vi "Lockin-4461_3.0.vi"(8 "stop":bool) -> (2 "Display 1X":dbl[](graph)=[5.429724320110079e-13, -1.0557648864671476e-12, -7.674396641294021e-14, -6.653872278941454e-13, 1.3512543311352937e-12, -8.695676182925118e-13, -1.9628415610324213e-13, -4.509112104711529e-13, -1.9014266708170094e-12, 5.798774579361177e-13, -8.609700256728925e-13, 7.075652959220096e-13, 9.045027478829498e-13, -6.452533894564113e-13, 4.967470274756812e-13, 8.424888248361009e-13, 6.406927601195649e-13, -8.489816114227698e-13, 1.1065735225780592e-12, -1.952661948744721e-12, -6.717167153798251e-13, 2.170352451318973e-12, 8.533633164810356e-13, 3.230898571625721e-08, 1.4746248954003764e-12, 1.3839944130800006e-12, -1.3057445582402538e-12, -5.535836882611926e-13, -3.127772440618251e-14, -5.486152818365045e-13, -6.837509468559333e-13, -1.101009850575611e-12, -8.217908360205046e-13, 1.5919674852128345e-13, -6.878154271851141e-13, 7.351033185025182e-13, 5.704450436053545e-13, -3.500521783374724e-13, -2.9031325786509e-13, 5.361241873731532e-13, 6.133239353042052e-13, -7.509096844850103e-13, -6.782070528277833e-13, 3.6986407984691915e-13, 1.2875981278874305e-12, -9.126571382818947e-13, -1.4081682222822822e-12, 6.601643304983332e-13, 3.358604874049834e-13, 6.17891015492966e-14, 7.388961275588427e-13, -3.190507233632056e-13, 6.464810882642673e-13, -1.0585784637759772e-12, 3.1545303767551145e-13, 8.8030129738905e-13, 1.899524086368318e-12, -1.0211002590514256e-12, -8.842995728059487e-13, 4.651074986030093e-13, 0.0, 0.0, 0.0, 0.0, 0.0, 0.0, 0.0, 0.0, 0.0, 0.0, 0.0, 0.0, 0.0, 0.0, 0.0, 0.0, 0.0, 0.0, 0.0, 0.0, 0.0, 0.0, 0.0, 0.0, 0.0, 0.0, 0.0, 0.0, 0.0, 0.0, 0.0, 0.0, 0.0, 0.0, 0.0, 0.0, 0.0, 0.0, 0.0, 0.0, 0.0, 0.0, 0.0, 0.0, 0.0, 0.0, 0.0, 0.0, 0.0, 0.0, 0.0, 0.0, 0.0, 0.0, 0.0, 0.0, 0.0, 0.0, 0.0, 0.0, 0.0, 0.0, 0.0, 0.0, 0.0, 0.0, 0.0, 0.0, 0.0, 0.0, 0.0, 0.0, 0.0, 0.0, 0.0, 0.0, 0.0, 0.0, 0.0, 0.0, 0.0, 0.0, 0.0, 0.0, 0.0, 0.0, 0.0, 0.0, 0.0, 0.0, 0.0, 0.0, 0.0, 0.0, 0.0, 0.0, 0.0, 0.0, 0.0, 0.0, 0.0, 0.0, 0.0, 0.0, 0.0, 0.0, 0.0, 0.0, 0.0, 0.0, 0.0, 0.0, 0.0, 0.0, 0.0, 0.0, 0.0, 0.0, 0.0, 0.0, 0.0, 0.0, 0.0, 0.0, 0.0, 0.0, 0.0, 0.0, 0.0, 0.0, 0.0, 0.0, 0.0, 0.0, 0.0, 0.0, 0.0, 0.0, 0.0, 0.0], 3 "Input signal":dbl[][](graph))   [LabVIEW 2011]
uses:
  <vilib>/DAQmx/write.llb/DAQmx Write (Analog 1D Wfm NChan NSamp).vi
  <vilib>/DAQmx/read.llb/DAQmx Read (Analog 2D DBL NChan NSamp).vi
  DAQ-lockin-SubVI/Source/Lock-in Globles.vi
  <vilib>/DAQmx/create/channels.llb/DAQmx Create Channel (AO-Voltage-Basic).vi
  <vilib>/DAQmx/configure/timing.llb/DAQmx Timing (Sample Clock).vi
  <vilib>/DAQmx/create/channels.llb/DAQmx Create Channel (AI-Voltage-Basic).vi
  <vilib>/DAQmx/configure/trigger.llb/DAQmx Start Trigger (Digital Edge).vi
  <vilib>/DAQmx/miscellaneous.llb/DAQmx Fill In Error Info.vi
  <vilib>/Analysis/2dsp.llb/Decimate (single shot, DBL).vi
  C:/Program Files (x86)/National Instruments/LabVIEW 2011/resource/objmgr/daqmx.rc
  <vilib>/Analysis/NI_AALPro.lvlib
  <vilib>/measure/NI_MABase.lvlib
panel:
  in  "Tab Control 2":T1(tab)
  in  "Auto control  max AI rate/ AI block size":bool=TRUE
  in  "AI Buffer Size (s)":i32=50
  in  "AI Block Size":i32=20000
  out "AI Rate":dbl=26920.0 format="%.2f"
  in  "AI Configuration":T2(array[cluster])=[{"AI.Coupling"=10050, "AI.Max"=10.0, "AI.Min"=-10.0, "Input physical channels"="PXI1Slot2/ai0:1"}, {"AI.Coupling"=10050, "AI.Max"=10.0, "AI.Min"=-10.0, "Input physical channels"="PXI1Slot3/ai0:1"}] {"AI.Coupling" items=["AC"=10045, "DC"=10050, "GND"=10066]}
  in  "AO Configuration":T3(array[cluster])=[{"Output physical channels"="PXI1Slot2/ao0:1", "AO. Max"=0.1, "AO.Min"=-0.1}, {"Output physical channels"="PXI1Slot3/ao0:1", "AO. Max"=0.1, "AO.Min"=-0.1}]
  in  "OSC Configuration":T4(array[cluster])=[{"Signal Type"=enum."Sine Wave", "DC"=0.0005, "Amplitude"=0.005, "frequency"=1.346, "Phase"=0.0}, {"Signal Type"=enum."Sine Wave", "DC"=0.0, "Amplitude"=0.0, "frequency"=1.346, "Phase"=0.0}, {"Signal Type"=enum."Sine Wave", "DC"=0.0, "Amplitude"=0.0, "frequency"=1.346, "Phase"=0.0}, {"Signal Type"=enum."Sine Wave", "DC"=0.0, "Amplitude"=0.0, "frequency"=1.346, "Phase"=0.0}] {"frequency" step=0.001 format="%.3p"; "Amplitude" format="%0.2p"; "DC" min=-0.99 max=0.99 format="%.2p"}
  in  "Phase&Tc":T5(array[cluster])=[{"Phase"=0.0, "Time constant"=0.1, "Set Tc"=FALSE, "Autophase"=FALSE, "Order"=2.0}, {"Phase"=0.0, "Time constant"=0.1, "Set Tc"=FALSE, "Autophase"=FALSE, "Order"=2.0}, {"Phase"=0.0, "Time constant"=0.1, "Set Tc"=FALSE, "Autophase"=FALSE, "Order"=2.0}, {"Phase"=0.0, "Time constant"=0.1, "Set Tc"=FALSE, "Autophase"=FALSE, "Order"=2.0}] {"Phase" min=0.0 max=360.0 scale=0.0..360.0}
  in  "Amplifier Settings":u16[](array[ring])=[0, 1, 2, 3] items=["DDPCA1", "DDPCA2", "DLPVA3", "DLPVA4"]
  out "Gains":dbl[](array[numeric])=[1000000.0, 10000.0, 100.0, 100.0]
  out "Display 2":string="-  1.764176      pA"
  out "Display 1":string=" 465.107499      fA"
  in  "Tab Control":T6(tab)=enum."Input signals"
  out "Display 1Y":dbl[](graph)=[-6.015136776726478e-13, 1.035472311764227e-12, 5.188198353772234e-13, 9.334164779082207e-14, -1.5030194120082668e-12, -8.299659830246285e-13, 5.929651298804293e-13, 1.4303475305665126e-12, 1.233410917595558e-13, -4.942128189633786e-13, -5.56641126205868e-14, -1.6075217488647061e-12, -1.3472295800498274e-13, -8.683381116120352e-13, -1.3801350908965668e-12, -1.579973320066605e-12, -5.359911294273503e-13, -2.83602775541613e-13, -1.388283326074415e-13, 2.241587836500851e-12, 1.015818909665972e-12, 1.2063259781645677e-12, -7.237492590732482e-13, -2.0089800684537727e-09, -5.72873903946076e-13, 9.667067330086395e-13, -2.2804413354213683e-13, 9.302118872846608e-13, -1.7473197459755622e-13, -5.49548652613498e-13, 9.153961719844722e-14, 1.5128757165450556e-12, -1.611847036715737e-12, 1.673036083421127e-13, 1.895919985144317e-13, -2.2589321538926073e-12, 9.153463078684243e-13, 2.332390292749605e-12, 1.5850725180362008e-12, -1.2395161770271868e-12, -1.8617257075369522e-12, 8.960246859996906e-13, -4.858869389193005e-13, 8.800808803791886e-13, 1.2523505072344644e-12, 2.3323855476977413e-12, 1.7142382752330603e-12, -1.8963340507897093e-12, 1.752869886311412e-13, -3.356413093784719e-13, 2.2656871916040576e-13, 1.0273329424492362e-12, -2.1535849626269848e-13, -8.008825638107896e-13, -7.074468145745153e-14, 2.4483654170431395e-13, 8.164120676180945e-13, -1.0926978964631754e-12, -5.216842010670745e-13, -1.7641762037163097e-12, 0.0, 0.0, 0.0, 0.0, 0.0, 0.0, 0.0, 0.0, 0.0, 0.0, 0.0, 0.0, 0.0, 0.0, 0.0, 0.0, 0.0, 0.0, 0.0, 0.0, 0.0, 0.0, 0.0, 0.0, 0.0, 0.0, 0.0, 0.0, 0.0, 0.0, 0.0, 0.0, 0.0, 0.0, 0.0, 0.0, 0.0, 0.0, 0.0, 0.0, 0.0, 0.0, 0.0, 0.0, 0.0, 0.0, 0.0, 0.0, 0.0, 0.0, 0.0, 0.0, 0.0, 0.0, 0.0, 0.0, 0.0, 0.0, 0.0, 0.0, 0.0, 0.0, 0.0, 0.0, 0.0, 0.0, 0.0, 0.0, 0.0, 0.0, 0.0, 0.0, 0.0, 0.0, 0.0, 0.0, 0.0, 0.0, 0.0, 0.0, 0.0, 0.0, 0.0, 0.0, 0.0, 0.0, 0.0, 0.0, 0.0, 0.0, 0.0, 0.0, 0.0, 0.0, 0.0, 0.0, 0.0, 0.0, 0.0, 0.0, 0.0, 0.0, 0.0, 0.0, 0.0, 0.0, 0.0, 0.0, 0.0, 0.0, 0.0, 0.0, 0.0, 0.0, 0.0, 0.0, 0.0, 0.0, 0.0, 0.0, 0.0, 0.0, 0.0, 0.0, 0.0, 0.0, 0.0, 0.0, 0.0, 0.0, 0.0, 0.0, 0.0, 0.0, 0.0, 0.0, 0.0, 0.0, 0.0, 0.0]
  out "Display 2Y":dbl[](graph)=[-6.05941549125348e-10, -1.1430340211264505e-10, 1.4926553931835592e-11, 1.50809116720554e-11, -2.01455613432856e-11, 2.2500663508188414e-10, -5.53750322011223e-11, -6.325220260727363e-11, 8.972686914309565e-11, -2.1675695268903223e-10, -9.319257292382553e-11, 1.3837564135013927e-10, 3.011851516936912e-11, -1.0972720971516426e-10, -1.7192768819908462e-10, 2.1187205561264862e-10, 1.9788207965441777e-10, -2.423720638237454e-11, -2.4682239326811696e-10, -1.9335970803307808e-10, 7.039230417281883e-11, 9.011350062257116e-11, -2.665249606640579e-10, -1.453917866253117e-07, -3.0864865233522615e-10, 2.2568328220655327e-11, -1.2760612434779825e-10, 1.7406875297242865e-10, -4.880057645786918e-11, -4.660274739851506e-11, 5.7934677183048936e-11, -1.272005485436437e-10, 8.868903467098303e-11, 7.631865938582677e-11, -1.5204222349177603e-10, 1.9443492736339234e-10, -2.2100622603667065e-10, -2.363955107876496e-10, 2.553251678563293e-11, -2.8250212646006297e-10, 1.1669743589404862e-11, 2.2238028971674755e-10, 2.136484065752661e-11, 1.682371445988206e-10, 1.1620525101317565e-10, -5.560771582752512e-11, 1.2104587980470587e-10, -5.20682135443474e-11, -8.156865511367845e-11, 8.10218105283791e-11, 3.289346118088131e-11, 1.1804160110274542e-10, -5.039858478435064e-12, -1.0278298256200302e-10, -3.7448450807439117e-10, 4.9424826507365526e-11, 5.43485642775191e-11, -5.139023835896488e-11, -1.677271234483857e-11, -9.992163832446762e-11, 0.0, 0.0, 0.0, 0.0, 0.0, 0.0, 0.0, 0.0, 0.0, 0.0, 0.0, 0.0, 0.0, 0.0, 0.0, 0.0, 0.0, 0.0, 0.0, 0.0, 0.0, 0.0, 0.0, 0.0, 0.0, 0.0, 0.0, 0.0, 0.0, 0.0, 0.0, 0.0, 0.0, 0.0, 0.0, 0.0, 0.0, 0.0, 0.0, 0.0, 0.0, 0.0, 0.0, 0.0, 0.0, 0.0, 0.0, 0.0, 0.0, 0.0, 0.0, 0.0, 0.0, 0.0, 0.0, 0.0, 0.0, 0.0, 0.0, 0.0, 0.0, 0.0, 0.0, 0.0, 0.0, 0.0, 0.0, 0.0, 0.0, 0.0, 0.0, 0.0, 0.0, 0.0, 0.0, 0.0, 0.0, 0.0, 0.0, 0.0, 0.0, 0.0, 0.0, 0.0, 0.0, 0.0, 0.0, 0.0, 0.0, 0.0, 0.0, 0.0, 0.0, 0.0, 0.0, 0.0, 0.0, 0.0, 0.0, 0.0, 0.0, 0.0, 0.0, 0.0, 0.0, 0.0, 0.0, 0.0, 0.0, 0.0, 0.0, 0.0, 0.0, 0.0, 0.0, 0.0, 0.0, 0.0, 0.0, 0.0, 0.0, 0.0, 0.0, 0.0, 0.0, 0.0, 0.0, 0.0, 0.0, 0.0, 0.0, 0.0, 0.0, 0.0, 0.0, 0.0, 0.0, 0.0, 0.0, 0.0]
  out "Display 2X":dbl[](graph)=[-5.209540983663562e-10, -1.5459993952257682e-10, 1.6134503412289663e-11, 5.874866305556756e-13, 1.8940414692414204e-10, -7.864880538635719e-11, -1.175430512415376e-10, -2.923449289922303e-11, -6.392419331917415e-11, -1.8337713666585666e-10, 1.378475926172313e-10, -2.033812689548571e-10, -4.8048021398079545e-11, 7.294621415013202e-11, -6.79053402284533e-11, -7.041661428266651e-11, -1.191656553793978e-10, -3.98775872041001e-11, 1.2696913609598267e-10, -2.604239565237904e-10, 2.421076799515798e-10, -9.586074443643207e-11, -2.670963844572135e-10, 2.3385861272623584e-06, -2.9864057097814606e-10, 4.050418120279296e-11, -8.73073671365595e-11, -2.2776227141712676e-10, 1.144251733636391e-10, 2.121387219366175e-10, 3.147413611980354e-11, -2.2045845902891772e-10, -9.974235087472864e-12, 5.4453485720179784e-11, 5.028348142025519e-11, -8.026581489308628e-11, -2.006232390289361e-10, -1.4683256880763738e-11, 1.2632039237668658e-10, -6.918201795183262e-11, 7.298099701633311e-11, 1.854494343744141e-10, -4.5058253262358714e-11, 6.898844457595054e-11, 1.3404894551663646e-10, -1.269804638347461e-10, -2.584513218696582e-10, -2.0850398617076455e-10, -1.1159639123537056e-11, -2.3248834236143404e-10, -2.1026006211792789e-10, 2.970246156973531e-10, -2.6985987935710656e-10, -1.0627514528789378e-10, -2.56461698957206e-10, -4.125165616305741e-11, -1.2485179826393064e-10, -4.1504869044150744e-11, 5.037294163088094e-11, 3.015780559703068e-11, 0.0, 0.0, 0.0, 0.0, 0.0, 0.0, 0.0, 0.0, 0.0, 0.0, 0.0, 0.0, 0.0, 0.0, 0.0, 0.0, 0.0, 0.0, 0.0, 0.0, 0.0, 0.0, 0.0, 0.0, 0.0, 0.0, 0.0, 0.0, 0.0, 0.0, 0.0, 0.0, 0.0, 0.0, 0.0, 0.0, 0.0, 0.0, 0.0, 0.0, 0.0, 0.0, 0.0, 0.0, 0.0, 0.0, 0.0, 0.0, 0.0, 0.0, 0.0, 0.0, 0.0, 0.0, 0.0, 0.0, 0.0, 0.0, 0.0, 0.0, 0.0, 0.0, 0.0, 0.0, 0.0, 0.0, 0.0, 0.0, 0.0, 0.0, 0.0, 0.0, 0.0, 0.0, 0.0, 0.0, 0.0, 0.0, 0.0, 0.0, 0.0, 0.0, 0.0, 0.0, 0.0, 0.0, 0.0, 0.0, 0.0, 0.0, 0.0, 0.0, 0.0, 0.0, 0.0, 0.0, 0.0, 0.0, 0.0, 0.0, 0.0, 0.0, 0.0, 0.0, 0.0, 0.0, 0.0, 0.0, 0.0, 0.0, 0.0, 0.0, 0.0, 0.0, 0.0, 0.0, 0.0, 0.0, 0.0, 0.0, 0.0, 0.0, 0.0, 0.0, 0.0, 0.0, 0.0, 0.0, 0.0, 0.0, 0.0, 0.0, 0.0, 0.0, 0.0, 0.0, 0.0, 0.0, 0.0, 0.0]
  out "Display 3Y":dbl[](graph)=[1.0899898431091515e-10, -1.827581519364685e-12, 3.891613088455869e-11, 4.606171792041084e-11, 3.325661502628918e-12, -6.015405048742651e-12, -8.818353730362106e-11, 4.154207587561132e-11, -6.441406967923057e-11, 2.7579642959096873e-11, 2.0247087826419377e-11, -8.327687150568863e-11, 5.645080566267779e-11, -6.157569018085951e-11, 1.1122174682043351e-11, -1.1996281757831183e-11, -2.6504845634178765e-11, -7.647423208254622e-11, 6.071533763218894e-11, -1.1261384601368719e-11, -1.0198381627901654e-11, 4.1339495592751516e-11, -1.5455592976820754e-11, 2.728948705870054e-08, 6.241263230606365e-11, -8.067722846760717e-11, -2.6513314314513534e-11, 6.394988304236903e-13, 3.9796667437030913e-13, 1.8692070371173484e-11, 9.340608297065955e-11, 2.3993660602172896e-11, -9.58560062287006e-11, 3.8126603558907844e-11, 1.1951601605204586e-10, 1.2004854916369822e-11, -8.43116466469951e-11, 4.536911918648911e-11, 8.587454567532404e-12, -5.1038971112404856e-11, 6.843278254393681e-11, -3.580011760107027e-12, -1.1591384728859565e-10, -5.389281317320638e-11, 2.0343389219590334e-11, -3.787714436214173e-11, -3.9748137155015685e-12, 5.264509352400637e-11, -2.982753663474114e-11, -3.4995836799112112e-12, -3.8221570403607076e-11, -4.7570393506646275e-11, 2.1951355761018474e-11, 2.0837341666890554e-11, -5.287022087117066e-11, 2.712528172281736e-11, 5.1245525962428926e-11, -6.547691762506247e-11, 1.5121870291068263e-12, -2.2769855527826617e-11, 0.0, 0.0, 0.0, 0.0, 0.0, 0.0, 0.0, 0.0, 0.0, 0.0, 0.0, 0.0, 0.0, 0.0, 0.0, 0.0, 0.0, 0.0, 0.0, 0.0, 0.0, 0.0, 0.0, 0.0, 0.0, 0.0, 0.0, 0.0, 0.0, 0.0, 0.0, 0.0, 0.0, 0.0, 0.0, 0.0, 0.0, 0.0, 0.0, 0.0, 0.0, 0.0, 0.0, 0.0, 0.0, 0.0, 0.0, 0.0, 0.0, 0.0, 0.0, 0.0, 0.0, 0.0, 0.0, 0.0, 0.0, 0.0, 0.0, 0.0, 0.0, 0.0, 0.0, 0.0, 0.0, 0.0, 0.0, 0.0, 0.0, 0.0, 0.0, 0.0, 0.0, 0.0, 0.0, 0.0, 0.0, 0.0, 0.0, 0.0, 0.0, 0.0, 0.0, 0.0, 0.0, 0.0, 0.0, 0.0, 0.0, 0.0, 0.0, 0.0, 0.0, 0.0, 0.0, 0.0, 0.0, 0.0, 0.0, 0.0, 0.0, 0.0, 0.0, 0.0, 0.0, 0.0, 0.0, 0.0, 0.0, 0.0, 0.0, 0.0, 0.0, 0.0, 0.0, 0.0, 0.0, 0.0, 0.0, 0.0, 0.0, 0.0, 0.0, 0.0, 0.0, 0.0, 0.0, 0.0, 0.0, 0.0, 0.0, 0.0, 0.0, 0.0, 0.0, 0.0, 0.0, 0.0, 0.0, 0.0]
  out "Display 3X":dbl[](graph)=[-1.4506921493871724e-12, -2.1744765834798285e-11, -3.886449186645477e-11, -7.085075187709098e-11, -3.9703339888141896e-11, 6.618132054310167e-11, -9.271260346821464e-12, 2.7348315791542174e-12, 3.091064650959652e-11, -1.3894193780750186e-11, 7.533626719542495e-11, -6.483103188230643e-11, -5.33856411786715e-11, -2.7467380020240738e-11, -6.103708902358562e-11, -2.2007178072058763e-11, 5.834941866531552e-11, 1.1615954777255411e-11, 8.406802135603188e-11, -4.803026535071808e-11, -2.3125249162347927e-11, 2.0152063097533814e-11, 1.6224115392482473e-11, -3.1111409147652163e-07, 7.799316159585665e-11, -1.1824501871462652e-10, -2.368710541907279e-11, 1.4150563678744927e-11, 5.694824941132326e-11, -9.713715348329474e-11, 2.3131114913051142e-11, -1.8619546897619826e-11, 1.9758889124328603e-11, 2.2778491607887418e-12, -4.1834293971028396e-11, -5.885822907793353e-11, -6.035522084307104e-12, 9.06513127169592e-11, 1.9006803683115078e-12, 3.2411130907631515e-11, -2.504571126204641e-11, -1.672617800966489e-11, -2.2621410052980212e-11, 2.8752008542406313e-11, 1.4141881559218766e-10, -6.022739594210222e-11, 1.4398026519979456e-12, 1.2286212124405088e-11, -8.788648695465874e-11, -3.125736625851777e-11, 6.67849549114717e-11, -6.608662073589525e-11, -1.6367174628356684e-12, -6.139681780409842e-11, 6.804379071422838e-11, -4.089900137250954e-11, -5.2810993260533214e-11, 8.44174959623023e-12, 3.1714297415210564e-11, -2.1731790500508637e-11, 0.0, 0.0, 0.0, 0.0, 0.0, 0.0, 0.0, 0.0, 0.0, 0.0, 0.0, 0.0, 0.0, 0.0, 0.0, 0.0, 0.0, 0.0, 0.0, 0.0, 0.0, 0.0, 0.0, 0.0, 0.0, 0.0, 0.0, 0.0, 0.0, 0.0, 0.0, 0.0, 0.0, 0.0, 0.0, 0.0, 0.0, 0.0, 0.0, 0.0, 0.0, 0.0, 0.0, 0.0, 0.0, 0.0, 0.0, 0.0, 0.0, 0.0, 0.0, 0.0, 0.0, 0.0, 0.0, 0.0, 0.0, 0.0, 0.0, 0.0, 0.0, 0.0, 0.0, 0.0, 0.0, 0.0, 0.0, 0.0, 0.0, 0.0, 0.0, 0.0, 0.0, 0.0, 0.0, 0.0, 0.0, 0.0, 0.0, 0.0, 0.0, 0.0, 0.0, 0.0, 0.0, 0.0, 0.0, 0.0, 0.0, 0.0, 0.0, 0.0, 0.0, 0.0, 0.0, 0.0, 0.0, 0.0, 0.0, 0.0, 0.0, 0.0, 0.0, 0.0, 0.0, 0.0, 0.0, 0.0, 0.0, 0.0, 0.0, 0.0, 0.0, 0.0, 0.0, 0.0, 0.0, 0.0, 0.0, 0.0, 0.0, 0.0, 0.0, 0.0, 0.0, 0.0, 0.0, 0.0, 0.0, 0.0, 0.0, 0.0, 0.0, 0.0, 0.0, 0.0, 0.0, 0.0, 0.0, 0.0]
  out "Display 4Y":dbl[](graph)=[-2.8844026407170986e-11, 4.625382034220138e-11, -9.013319110948715e-11, -3.831386252102219e-11, 2.9770810866125426e-11, -1.1034670821175042e-10, 1.5257307046567804e-11, 4.8262499387874416e-11, 1.3544857909536598e-11, 1.856703050862052e-13, 2.5150436114529384e-11, -2.094748767689225e-11, -7.22408300489974e-11, -1.6319787062002432e-11, -2.6839509106935107e-11, -6.340509375775128e-11, -2.7129427161298733e-11, 4.060501667453309e-11, 8.742730286854794e-11, -7.855807339041121e-11, 3.2402653147300955e-12, -3.7221693179390055e-11, -2.721498060225258e-11, 3.163166146765944e-08, 1.9865867500357126e-11, 3.370069404127207e-11, -2.1485622596628672e-11, -1.086161315512868e-10, -1.5918432616501835e-11, -8.641508247819728e-12, -3.272966578151681e-11, -3.9968869914730473e-11, -3.7871727870708584e-11, 1.782636420557537e-11, -4.727645885793663e-12, -3.739448916633137e-11, 2.2633565117757826e-11, 3.480934154822535e-11, 7.660374794795644e-11, 4.2421105834478115e-11, -4.7175325158832496e-11, 7.467358811652501e-12, 9.053400661116483e-11, 7.680172474522351e-11, 1.9234239962884202e-11, -4.05154145894926e-11, 1.0289905284821542e-11, 1.026100591445811e-11, 2.583088099896713e-11, 4.907786066752351e-11, 5.609058148507984e-11, -3.1281978648678434e-11, -2.3787541867648086e-11, 2.931160232435559e-11, -4.803534531703235e-11, 8.40306343263819e-11, -4.556520949563492e-11, 2.7403738536690982e-11, 6.669893713819875e-11, -2.2080502155574778e-11, 0.0, 0.0, 0.0, 0.0, 0.0, 0.0, 0.0, 0.0, 0.0, 0.0, 0.0, 0.0, 0.0, 0.0, 0.0, 0.0, 0.0, 0.0, 0.0, 0.0, 0.0, 0.0, 0.0, 0.0, 0.0, 0.0, 0.0, 0.0, 0.0, 0.0, 0.0, 0.0, 0.0, 0.0, 0.0, 0.0, 0.0, 0.0, 0.0, 0.0, 0.0, 0.0, 0.0, 0.0, 0.0, 0.0, 0.0, 0.0, 0.0, 0.0, 0.0, 0.0, 0.0, 0.0, 0.0, 0.0, 0.0, 0.0, 0.0, 0.0, 0.0, 0.0, 0.0, 0.0, 0.0, 0.0, 0.0, 0.0, 0.0, 0.0, 0.0, 0.0, 0.0, 0.0, 0.0, 0.0, 0.0, 0.0, 0.0, 0.0, 0.0, 0.0, 0.0, 0.0, 0.0, 0.0, 0.0, 0.0, 0.0, 0.0, 0.0, 0.0, 0.0, 0.0, 0.0, 0.0, 0.0, 0.0, 0.0, 0.0, 0.0, 0.0, 0.0, 0.0, 0.0, 0.0, 0.0, 0.0, 0.0, 0.0, 0.0, 0.0, 0.0, 0.0, 0.0, 0.0, 0.0, 0.0, 0.0, 0.0, 0.0, 0.0, 0.0, 0.0, 0.0, 0.0, 0.0, 0.0, 0.0, 0.0, 0.0, 0.0, 0.0, 0.0, 0.0, 0.0, 0.0, 0.0, 0.0, 0.0]
  out "Display 4X":dbl[](graph)=[-1.872849874212032e-11, 1.7122412246892844e-11, -1.039280965881989e-11, -3.8219137836769534e-11, 2.54510636198968e-12, 5.649551705638675e-11, -1.2837219048125736e-11, 6.089320247177828e-11, 8.191453420346272e-12, -2.2600834935992963e-11, -5.439952919719105e-11, 5.769571050429079e-11, 1.9308897762471135e-11, -3.4192678553779385e-11, 9.300946324977131e-11, -1.727038806027537e-11, 7.995920408632173e-12, 4.071400274554549e-11, 2.268153369371362e-11, -2.0174647879223076e-11, 1.0691363677679532e-10, -1.4886887784193447e-11, -5.66145435172416e-11, -3.1370210865590164e-07, 3.490142592397077e-11, -4.99211179772148e-11, 1.3636252598244609e-11, 3.3098859041298666e-12, -1.6672726161063438e-11, 1.4892486798539355e-11, 5.223389085892288e-11, 1.9716195076308757e-11, -6.274884038088292e-11, 3.5321483840811124e-11, -7.835323866883167e-11, 1.2109030814600604e-11, 5.256527515492618e-11, 7.655498412083988e-12, -9.897929289071003e-11, 3.822872610482336e-12, 1.1209679192923232e-10, 2.9926432039962396e-11, 1.3077089526049997e-11, -4.870241767356217e-11, 2.5349979762609446e-11, 3.4612212078481696e-11, -7.616485687473168e-11, 1.7187008086182176e-11, 3.640759205650324e-12, 5.822438037809061e-11, 5.999925879620962e-11, -2.884252381395239e-11, 1.4931791499632476e-12, 2.5243703206574706e-11, -1.236460355930176e-10, 4.641707430741368e-11, -2.9998695243557e-11, -2.6680922547736572e-11, 1.4569031712088202e-11, 3.4952487260758724e-11, 0.0, 0.0, 0.0, 0.0, 0.0, 0.0, 0.0, 0.0, 0.0, 0.0, 0.0, 0.0, 0.0, 0.0, 0.0, 0.0, 0.0, 0.0, 0.0, 0.0, 0.0, 0.0, 0.0, 0.0, 0.0, 0.0, 0.0, 0.0, 0.0, 0.0, 0.0, 0.0, 0.0, 0.0, 0.0, 0.0, 0.0, 0.0, 0.0, 0.0, 0.0, 0.0, 0.0, 0.0, 0.0, 0.0, 0.0, 0.0, 0.0, 0.0, 0.0, 0.0, 0.0, 0.0, 0.0, 0.0, 0.0, 0.0, 0.0, 0.0, 0.0, 0.0, 0.0, 0.0, 0.0, 0.0, 0.0, 0.0, 0.0, 0.0, 0.0, 0.0, 0.0, 0.0, 0.0, 0.0, 0.0, 0.0, 0.0, 0.0, 0.0, 0.0, 0.0, 0.0, 0.0, 0.0, 0.0, 0.0, 0.0, 0.0, 0.0, 0.0, 0.0, 0.0, 0.0, 0.0, 0.0, 0.0, 0.0, 0.0, 0.0, 0.0, 0.0, 0.0, 0.0, 0.0, 0.0, 0.0, 0.0, 0.0, 0.0, 0.0, 0.0, 0.0, 0.0, 0.0, 0.0, 0.0, 0.0, 0.0, 0.0, 0.0, 0.0, 0.0, 0.0, 0.0, 0.0, 0.0, 0.0, 0.0, 0.0, 0.0, 0.0, 0.0, 0.0, 0.0, 0.0, 0.0, 0.0, 0.0]
  in  "Stream to disk?":bool
  in  "decimating factor":i32=400
  out "phase log":dbl[](array[numeric])=[0.999999999996331, 0.999999999996331, 0.999999999996331, 0.999999999996331]
  in  "Cancel Button":bool
  in  "Display":u16(ring) items=["X and Y", "R and Theta"]
  out "Results":dbl[][](array[numeric])=[[4.6510749860300926e-07, -1.7641762037163097e-06, 1.8244568131407326e-06, -75.23060410302357], [3.015780559703068e-07, -9.992163832446762e-07, 1.043734978041553e-06, -73.20542108368687], [-2.1731790500508636e-09, -2.276985552782662e-09, 3.147597558640707e-09, -133.6637356996649], [3.4952487260758724e-09, -2.208050215557478e-09, 4.134277374772819e-09, -32.28179248079797]]
  out "Backlog":u8(slide) scale=0.0..100.0
  out "Sampling information":cluster{"Fs":dbl, "#s":dbl}[](array[cluster])=[{"Fs"=26920.0, "#s"=20000.0}, {"Fs"=26920.0, "#s"=20000.0}]
  out "AO Task":refnum<k21>[](array[refnum])
  out "AI task":refnum<k21>[](array[refnum])
  out "Signal":dbl[][](array[numeric])
  # "Real time Adjustable Values"
  # "Configurations"
  # "Features:\n1, up to 4 lock-in amplifiers\n2, Each AO outputs an DC+AC signal, DC for sample biasing and AC for OSC. These values can be adjusted in real time.\n3, Synchronous filtering\n\nInstructions:\n1, Array index of AI configuration and AO configuration referes to board number. We have 2 PXI-4461 boards, so the max index is 1.\n2, Array number OSC configuration, Phase$&Tc control correlates to lock-in #., max index is 4.\n3, Each board can have 2 lock-in channels. Syntax for 2 channles, e.g. PXI1Slot2/ai0:1. If you want to use just one, then PXI1Slot2/ai0.\n4, Parameters (especially DC value for sample biasing) can be remotely controlled by clicking \"local\"and \"remote\" button. In real experiments, put golable values (can be found in Lock-in globles.vi) in your VI to control the lock-in and read out.\n5, choose OSC frequencies to be multiple of \nAI Rate/AI Block SIze to have best performance.\n\n-Guanglei 06/23/2011"
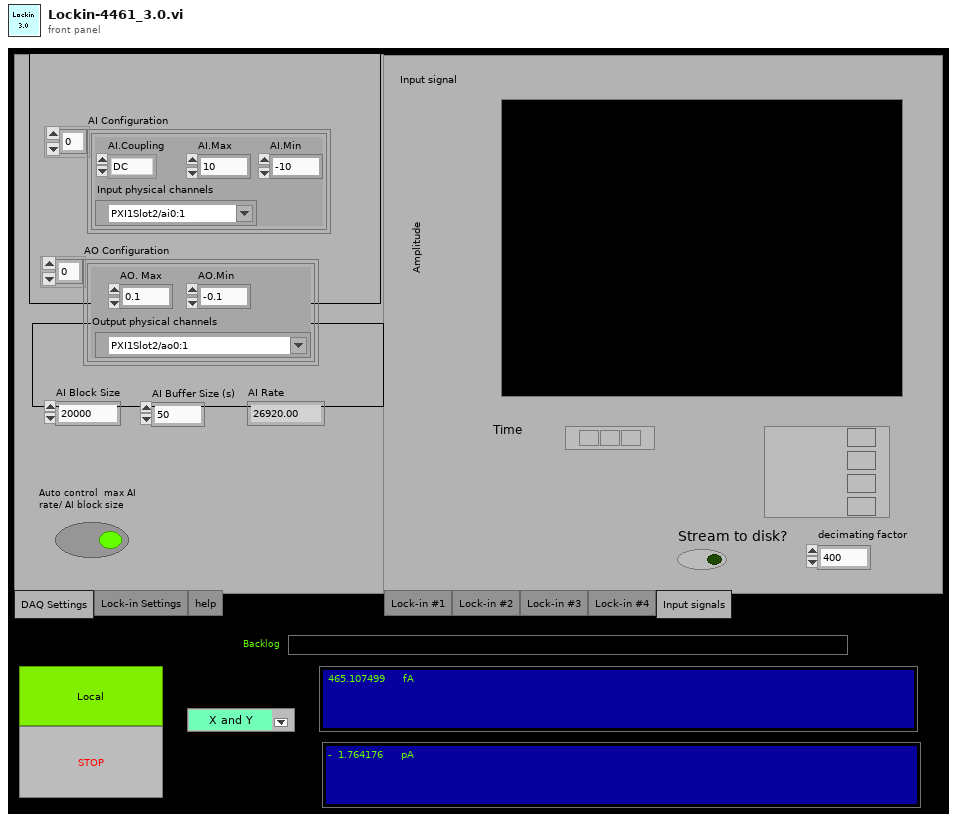
[diagram p1: front panel]
types:
  T1 = enum32{"DAQ Settings", "Lock-in Settings", "help"}
  T2 = cluster{"AI.Coupling":i32, "AI.Max":dbl, "AI.Min":dbl, "Input physical channels":tag}[]
  T3 = cluster{"Output physical channels":tag, "AO. Max":dbl, "AO.Min":dbl}[]
  T4 = cluster{"Signal Type":enum16{"Sine Wave", "Triangle Wave", "Square Wave", "Sawtooth Wave"}, "DC":dbl, "Amplitude":dbl, "frequency":dbl, "Phase":dbl}[]
  T5 = cluster{"Phase":dbl, "Time constant":dbl, "Set Tc":bool, "Autophase":bool, "Order":dbl}[]
  T6 = enum32{"Lock-in #1", "Lock-in #2", "Lock-in #3", "Lock-in #4", "Input signals"}
  T7 = cluster{"Signal Type":enum16{"Sine Wave", "Triangle Wave", "Square Wave", "Sawtooth Wave"}, "DC":dbl, "Amplitude":dbl, "frequency":dbl, "Phase":dbl}
  T8 = cluster{"AI.Coupling":i32, "AI.Max":dbl, "AI.Min":dbl, "Input physical channels":tag}
  T9 = cluster{"Output physical channels":tag, "AO. Max":dbl, "AO.Min":dbl}
  T10 = enum16{"Sine Wave", "Triangle Wave", "Square Wave", "Sawtooth Wave"}
  T11 = cluster{"Signal Type":u16, "DC":dbl, "Amplitude":dbl, "frequency":dbl, "Phase":dbl}[]
  T12 = cluster{"Signal Type":u16, "DC":dbl, "Amplitude":dbl, "frequency":dbl, "Phase":dbl}
  T13 = cluster{"Ref X":dbl[], "Ref Y":dbl[], "AI Rate":dbl, "AI Block Size":dbl, "Frequency":dbl, "Ref amp":dbl}
  T14 = cluster{"Phase":dbl, "Time constant":dbl, "Set Tc":bool, "Autophase":bool, "Order":dbl}
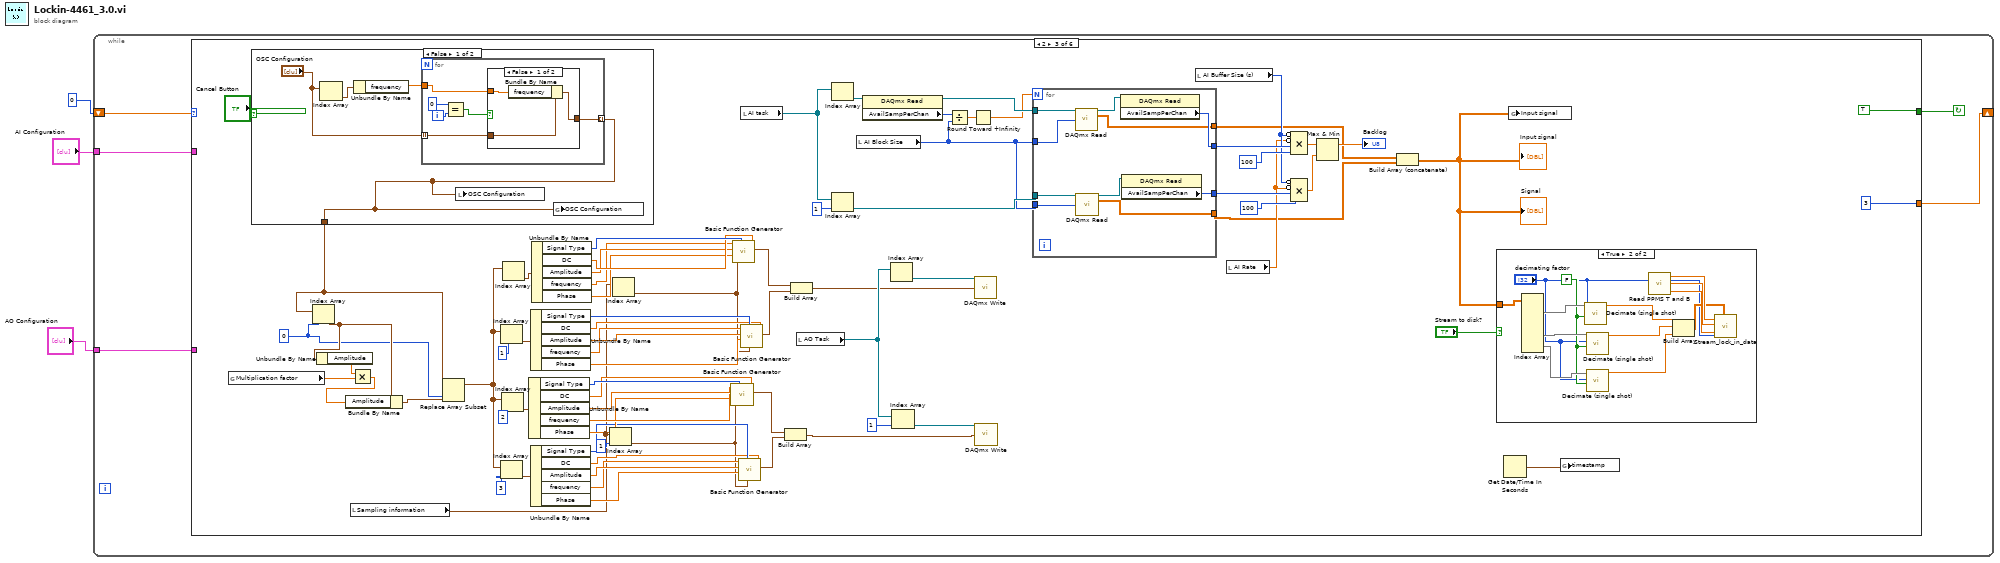
[diagram p0: block diagram]
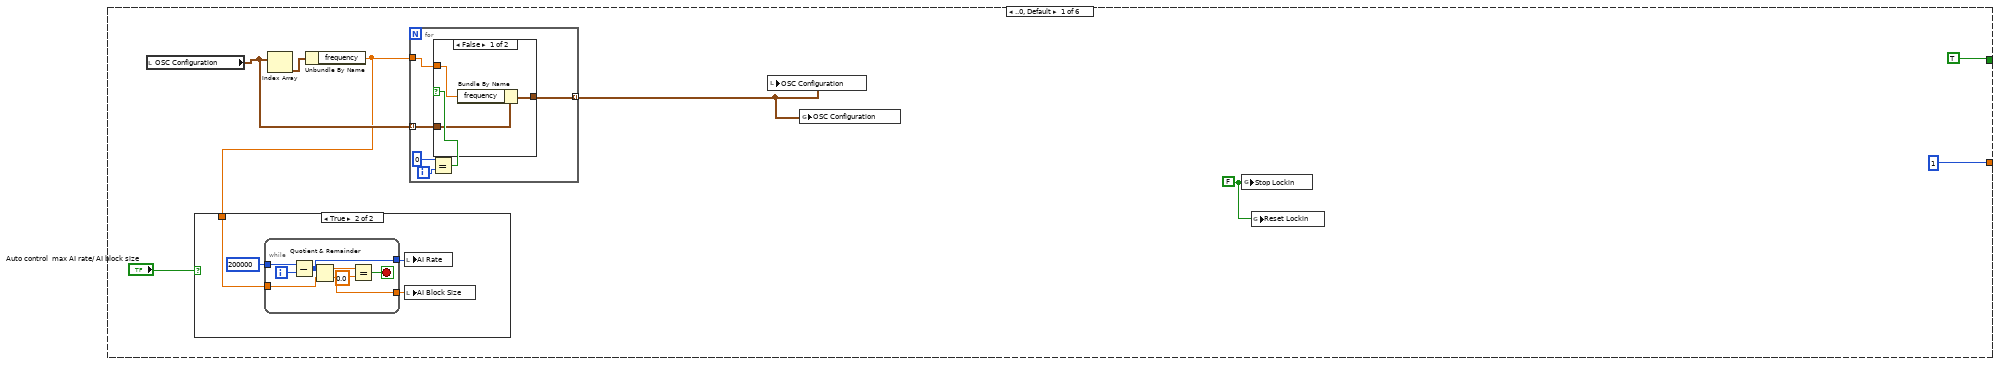
[diagram p2: hidden frame]
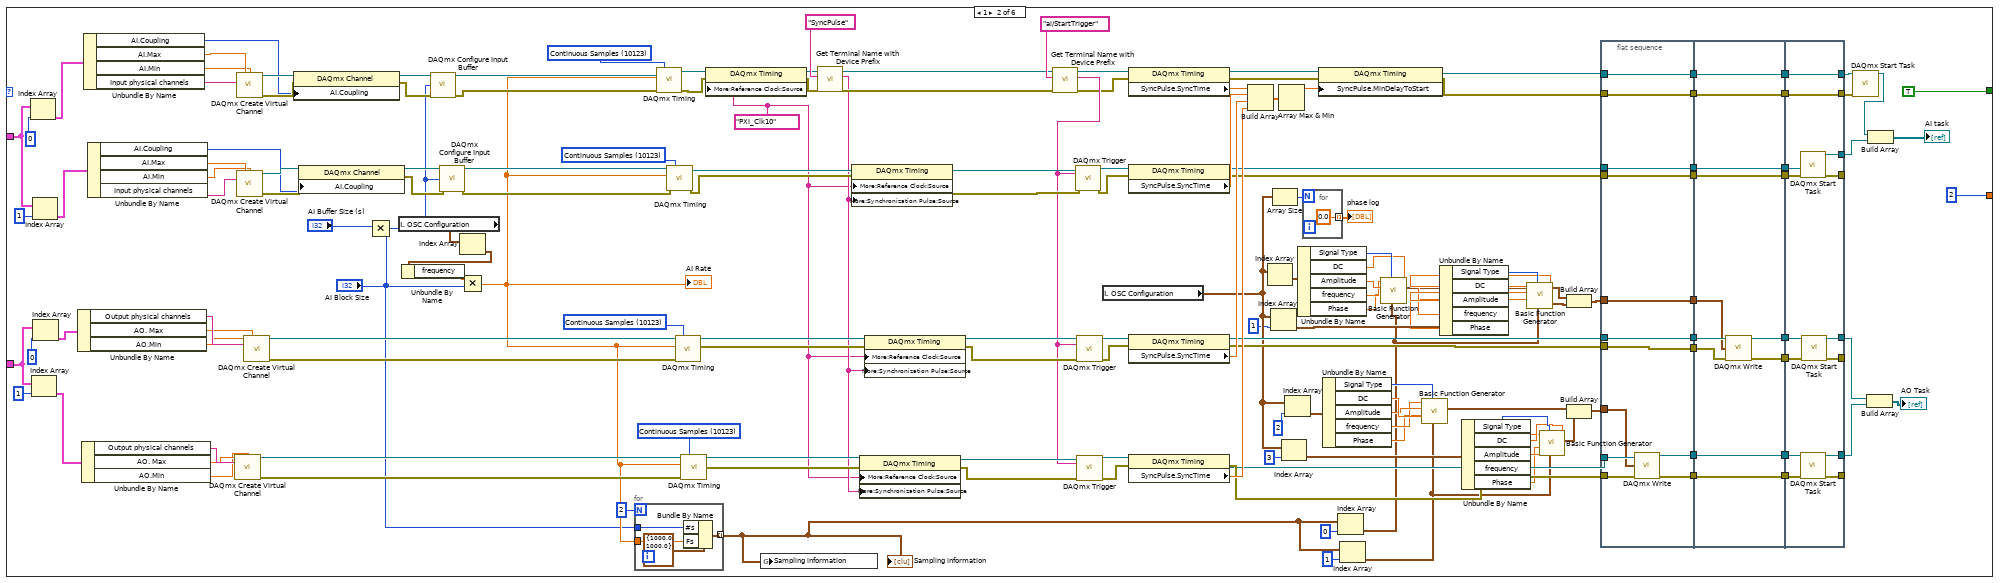
[diagram p5: hidden frame]
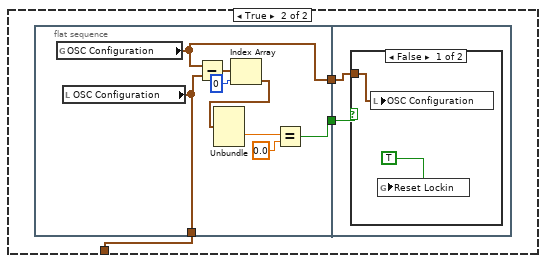
[diagram p8: hidden frame]
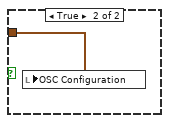
[diagram p9: hidden frame]
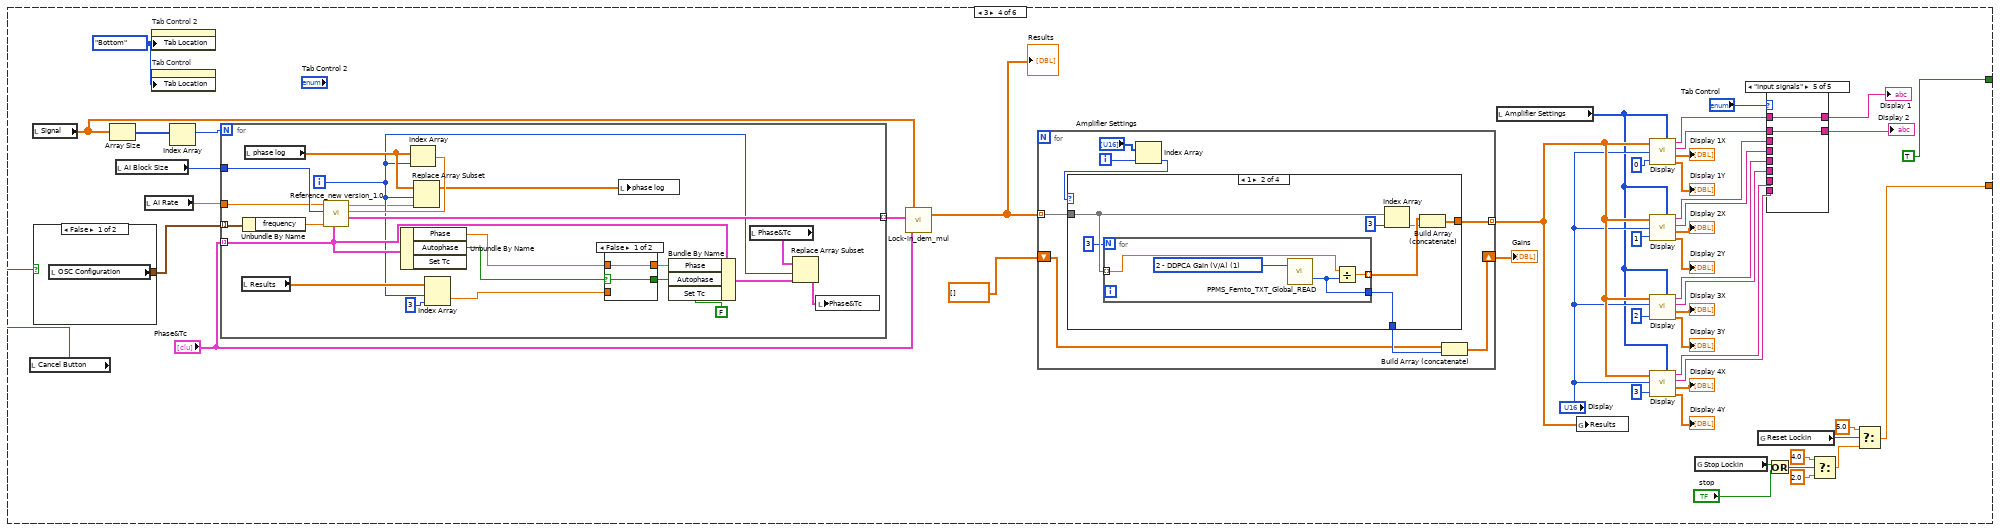
[diagram p10: hidden frame]
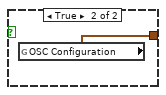
[diagram p11: hidden frame]
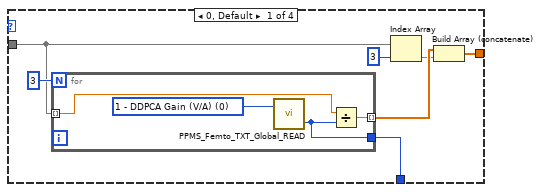
[diagram p16: hidden frame]
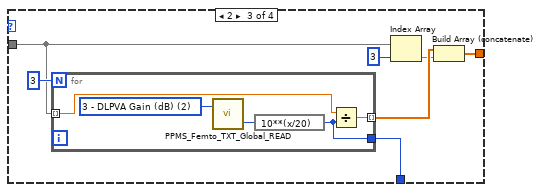
[diagram p17: hidden frame]
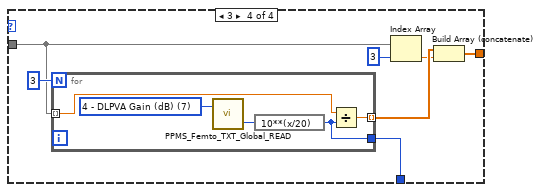
[diagram p18: hidden frame]
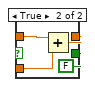
[diagram p19: hidden frame]
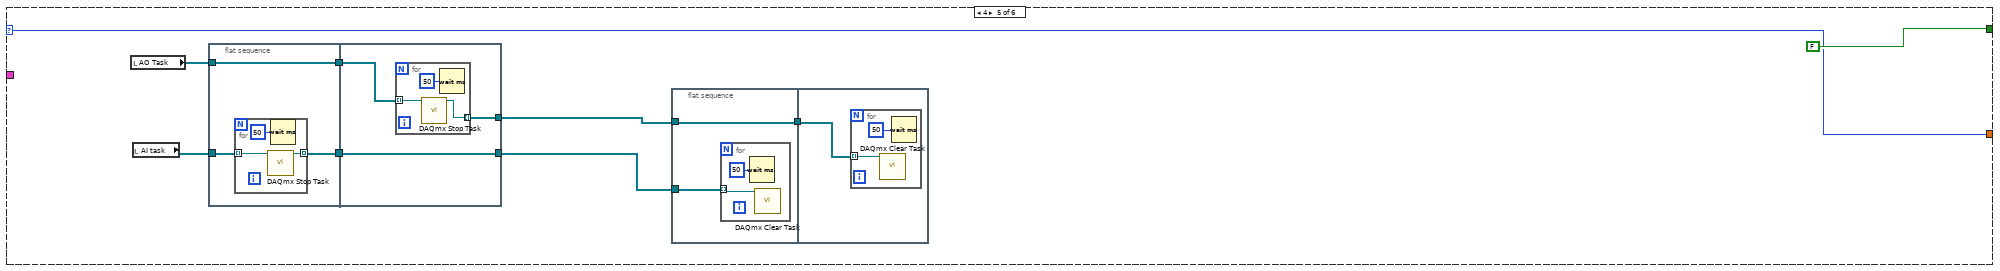
[diagram p20: hidden frame]
diagram:
  n1 = while {
    shift-right: [w8] -> _
    shift-left: 0 -> [w7]
    tunnel: "AI Configuration" -> [w6]
    tunnel: "AO Configuration" -> [w5]
    stop <- w4 continue-if-true
    n2 = case shown="2" w7 {
      selector: w7 -> [_ _ _ _ w526 _]
      tunnel: [1 2 3 w379 w526 0.0 ("f")] -> w8
      tunnel: w6 -> [_ w201 _ _ _ _]
      tunnel: w5 -> [_ w200 _ _ _ _]
      tunnel: [TRUE TRUE TRUE TRUE FALSE TRUE] -> w4
      frame ..0, Default {
        w14 = FALSE ("Stop Lockin")
        n3 = local read "OSC Configuration"() -> (w12:T4)
        n4 = Index Array(array=w12) -> (element=w13:T7)  [unwired: 1 in]
        n5 = Unbundle By Name(w13) -> ("frequency"=w11:dbl)
        n6 = case shown="True" "Auto control  max AI rate/ AI block size" {
          tunnel: w11 -> [_ w19]
          frame False {
          }
          frame True {
            n7 = while {
              tunnel: 200000 -> [w28]
              tunnel: w19 -> [w26]
              tunnel: [w22] -> w18
              tunnel: [w21] -> w17
              i -> [w27]
              stop <- w23 stop-if-true
              n8 = Subtract(x=w28, y=w27) -> (x-y=w21:i32)
              n9 = Quotient & Remainder(x=w21, y=w26) -> (x-y*floor(x/y)=w25:dbl, floor(x/y)=w22:dbl)
              n10 = Equal?(x=w25, y=0.0) -> (x = y?=w23:bool)
            }
            n11 = local write "AI Rate"(w17) -> ()
            n12 = local write "AI Block Size"(w18) -> ()
          }
        }
        n13 = for {
          tunnel: w12 -> [w31] mode=indexing
          tunnel: w11 -> [w30]
          tunnel: [w29] -> w9 mode=indexing
          i -> [w34]
          n14 = Equal?(x=0, y=w34) -> (x = y?=w32:bool)
          n15 = case shown="False" w32 {
            tunnel: w31 -> [w37 w38]
            tunnel: w30 -> [w36 _]
            tunnel: [w35 w38] -> w29
            frame False {
              n16 = Bundle By Name(cluster=w37, "frequency"=w36) -> (w35:T7)
            }
            frame True {
            }
          }
        }
        n17 = local write "OSC Configuration"(w9) -> ()
        n18 = global write "Lock-in Globles.vi" "OSC Configuration"(w9) -> ()
        n19 = global write "Lock-in Globles.vi" "Stop Lockin"(w14) -> ()
        n20 = global write "Lock-in Globles.vi" "Reset Lockin"(w14) -> ()
      }
      frame 1 {
        w108 = tag "PXI_Clk10" ("RefClk.Src")
        w166 = 10123 items=["Finite Samples"=10178, "Continuous Samples"=10123] ("sample mode")
        w167 = 10123 items=["Finite Samples"=10178, "Continuous Samples"=10123] ("sample mode")
        w174 = 10123 items=["Finite Samples"=10178, "Continuous Samples"=10123] ("sample mode")
        w175 = 10123 items=["Finite Samples"=10178, "Continuous Samples"=10123] ("sample mode")
        n21 = Index Array(array=w201, index=0) -> (element=w195:T8)
        n22 = Index Array(array=w200, index=1) -> (element=w193:T9)
        n23 = Index Array(array=w201, index=1) -> (element=w194:T8)
        n24 = Index Array(array=w200, index=0) -> (element=w192:T9)
        n25 = Unbundle By Name(w192) -> ("Output physical channels"=w117:tag, "AO. Max"=w116:dbl, "AO.Min"=w115:dbl)
        n26 = Unbundle By Name(w193) -> ("Output physical channels"=w114:tag, "AO. Max"=w113:dbl, "AO.Min"=w112:dbl)
        n27 = Unbundle By Name(w195) -> ("AI.Coupling"=w102:i32, "AI.Max"=w122:dbl, "AI.Min"=w121:dbl, "Input physical channels"=w123:tag)
        n28 = Unbundle By Name(w194) -> ("AI.Coupling"=w101:i32, "AI.Max"=w119:dbl, "AI.Min"=w118:dbl, "Input physical channels"=w120:tag)
        n29 = call-poly <vilib>:"DAQmx Create Virtual Channel.vi"("maximum value"=w113, "minimum value"=w112, "physical channels"=w114) -> ("task out"=w165:refnum<k21>, "error out"=w164:errorcluster)  [unwired: 11 in]
        n30 = call-poly <vilib>:"DAQmx Create Virtual Channel.vi"("maximum value"=w122, "minimum value"=w121, "physical channels"=w123) -> ("task out"=w106:refnum<k21>, "error out"=w105:errorcluster)  [unwired: 11 in]
        n31 = call-poly <vilib>:"DAQmx Create Virtual Channel.vi"("maximum value"=w119, "minimum value"=w118, "physical channels"=w120) -> ("task out"=w104:refnum<k21>, "error out"=w103:errorcluster)  [unwired: 11 in]
        n32 = call-poly <vilib>:"DAQmx Create Virtual Channel.vi"("maximum value"=w116, "minimum value"=w115, "physical channels"=w117) -> ("task out"=w125:refnum<k21>, "error out"=w124:errorcluster)  [unwired: 11 in]
        n33 = property class="DAQmx Channel"(reference=w106, error in=w105, "AI.Coupling"=w102) -> (reference out=w100:refnum<k21>, error out=w99:errorcluster)
        n34 = property class="DAQmx Channel"(reference=w104, error in=w103, "AI.Coupling"=w101) -> (reference out=w98:refnum<k21>, error out=w97:errorcluster)
        n35 = Multiply(x="AI Buffer Size (s)", y="AI Block Size") -> (x*y=w92:i32)
        n36 = local read "OSC Configuration"() -> (w46:T4)
        n37 = call <vilib>:"DAQmx Configure Input Buffer.vi"("task/channels in"=w100, "buffer size (in samples per channel)"=w92, "error in"=w99) -> ("task out"=w96:refnum<k21>, "error out"=w95:errorcluster)  [unwired: 11 in]
        n38 = call <vilib>:"DAQmx Configure Input Buffer.vi"("task/channels in"=w98, "buffer size (in samples per channel)"=w92, "error in"=w97) -> ("task out"=w94:refnum<k21>, "error out"=w93:errorcluster)  [unwired: 11 in]
        n39 = Index Array(array=w46) -> (element=w45:T7)  [unwired: 1 in]
        n40 = Unbundle By Name(w45) -> ("frequency"=w42:dbl)
        n41 = Multiply(x=w42, y="AI Block Size") -> (x*y=w44:dbl)
        "AI Rate" <- w44
        n42 = for {
          N: 2 -> [_]
          tunnel: w44 -> [w209]
          tunnel: "AI Block Size" -> [w208]
          tunnel: [w206] -> w64 mode=indexing
          n43 = Bundle By Name(cluster=cluster{"Fs":dbl, "#s":dbl} {"Fs"=1000.0, "#s"=1000.0} ("sampling info"), "#s"=w208, "Fs"=w209) -> (w206:cluster{"Fs":dbl, "#s":dbl})
        }
        "Sampling information" <- w64
        n44 = call-poly <vilib>:"DAQmx Timing.vi"("task/channels in"=w96, "sample mode"=w175, "rate"=w44, "error in"=w95) -> ("task out"=w169:refnum<k21>, "error out"=w168:errorcluster)  [unwired: 10 in]
        n45 = call-poly <vilib>:"DAQmx Timing.vi"("task/channels in"=w94, "sample mode"=w174, "rate"=w44, "error in"=w93) -> ("task out"=w171:refnum<k21>, "error out"=w170:errorcluster)  [unwired: 10 in]
        n46 = call-poly <vilib>:"DAQmx Timing.vi"("task/channels in"=w125, "sample mode"=w167, "rate"=w44, "error in"=w124) -> ("task out"=w162:refnum<k21>, "error out"=w161:errorcluster)  [unwired: 10 in]
        n47 = call-poly <vilib>:"DAQmx Timing.vi"("task/channels in"=w165, "sample mode"=w166, "rate"=w44, "error in"=w164) -> ("task out"=w163:refnum<k21>, "error out"=w158:errorcluster)  [unwired: 10 in]
        n48 = property class="DAQmx Timing"(reference=w169, error in=w168, "More:Reference Clock:Source"=w108) -> (reference out=w109:refnum<k21>, error out=w107:errorcluster)
        n49 = global write "Lock-in Globles.vi" "Sampling information"(w64) -> ()
        n50 = call "Get Terminal Name with Device Prefix.vi"("error in (no error)"=w107, "Local Terminal Name"="SyncPulse", "task/channels in"=w109) -> ("error out"=w151:errorcluster, "Terminal Name with Device Prefix"=w110:tag, "task out"=w152:refnum<k21>)  [unwired: 6 in]
        n51 = property class="DAQmx Timing"(reference=w171, error in=w170, "More:Reference Clock:Source"=w108, "More:Synchronization Pulse:Source"=w110) -> (reference out=w173:refnum<k21>, error out=w172:errorcluster)
        n52 = property class="DAQmx Timing"(reference=w163, error in=w158, "More:Reference Clock:Source"=w108, "More:Synchronization Pulse:Source"=w110) -> (reference out=w155:refnum<k21>, error out=w154:errorcluster)
        n53 = property class="DAQmx Timing"(reference=w162, error in=w161, "More:Reference Clock:Source"=w108, "More:Synchronization Pulse:Source"=w110) -> (reference out=w157:refnum<k21>, error out=w156:errorcluster)
        n54 = call "Get Terminal Name with Device Prefix.vi"("error in (no error)"=w151, "Local Terminal Name"="ai/StartTrigger", "task/channels in"=w152) -> ("error out"=w148:errorcluster, "Terminal Name with Device Prefix"=w150:tag, "task out"=w149:refnum<k21>)  [unwired: 6 in]
        n55 = call-poly <vilib>:"DAQmx Trigger.vi"("task/channels in"=w173, "source"=w150, "error in"=w172) -> ("task out"=w144:refnum<k21>, "error out"=w145:errorcluster)  [unwired: 11 in]
        n56 = call-poly <vilib>:"DAQmx Trigger.vi"("task/channels in"=w157, "source"=w150, "error in"=w156) -> ("task out"=w142:refnum<k21>, "error out"=w143:errorcluster)  [unwired: 11 in]
        n57 = call-poly <vilib>:"DAQmx Trigger.vi"("task/channels in"=w155, "source"=w150, "error in"=w154) -> ("task out"=w147:refnum<k21>, "error out"=w146:errorcluster)  [unwired: 11 in]
        n58 = local read "OSC Configuration"() -> (w65:T4)
        n59 = property class="DAQmx Timing"(reference=w149, error in=w148) -> (reference out=w139:refnum<k21>, error out=w140:errorcluster, "SyncPulse.SyncTime"=w141:dbl)
        n60 = property class="DAQmx Timing"(reference=w144, error in=w145) -> (reference out=w130:refnum<k21>, error out=w131:errorcluster, "SyncPulse.SyncTime"=w136:dbl)
        n61 = property class="DAQmx Timing"(reference=w142, error in=w143) -> (reference out=w128:refnum<k21>, error out=w129:errorcluster, "SyncPulse.SyncTime"=w135:dbl)
        n62 = property class="DAQmx Timing"(reference=w147, error in=w146) -> (reference out=w126:refnum<k21>, error out=w127:errorcluster, "SyncPulse.SyncTime"=w134:dbl)
        n63 = Build Array(w141, w136, w135, w134) -> (w138:dbl[])
        n64 = Index Array(array=w65) -> (element=w88:T7)  [unwired: 1 in]
        n65 = Index Array(array=w65, index=1) -> (element=w87:T7)
        n66 = Array Size(array=w65) -> (size(s)=w202:i32)
        n67 = Array Max & Min(array=w138) -> (max value=w137:dbl)  [unwired: 3 out]
        n68 = Index Array(array=w65, index=3) -> (element=w86:T7)
        n69 = Index Array(array=w65, index=2) -> (element=w89:T7)
        n70 = Unbundle By Name(w88) -> ("Signal Type"=w85:T10, "DC"=w84:dbl, "Amplitude"=w83:dbl, "frequency"=w82:dbl, "Phase"=w81:dbl)
        n71 = for {
          N: w202 -> [_]
          tunnel: [0.0] -> w203 mode=indexing
        }
        "phase log" <- w203
        n72 = property class="DAQmx Timing"(reference=w139, error in=w140, "SyncPulse.MinDelayToStart"=w137) -> (reference out=w132:refnum<k21>, error out=w133:errorcluster)
        n73 = Unbundle By Name(w89) -> ("Signal Type"=w75:T10, "DC"=w74:dbl, "Amplitude"=w73:dbl, "frequency"=w72:dbl, "Phase"=w71:dbl)
        n74 = Index Array(array=w64, index=0) -> (element=w61:cluster{"Fs":dbl, "#s":dbl})
        n75 = Index Array(array=w64, index=1) -> (element=w60:cluster{"Fs":dbl, "#s":dbl})
        n76 = call <vilib>:"Basic Function Generator.vi"("offset"=w84, "sampling info"=w61, "signal type"=w85, "phase"=w81, "amplitude"=w83, "frequency"=w82) -> ("signal out"=w59:waveform(dbl))  [unwired: 3 in, 2 out]
        n77 = call <vilib>:"Basic Function Generator.vi"("offset"=w74, "sampling info"=w60, "signal type"=w75, "phase"=w71, "amplitude"=w73, "frequency"=w72) -> ("signal out"=w55:waveform(dbl))  [unwired: 3 in, 2 out]
        n78 = Unbundle By Name(w87) -> ("Signal Type"=w80:T10, "DC"=w79:dbl, "Amplitude"=w78:dbl, "frequency"=w77:dbl, "Phase"=w76:dbl)
        n79 = Unbundle By Name(w86) -> ("Signal Type"=w70:T10, "DC"=w69:dbl, "Amplitude"=w68:dbl, "frequency"=w67:dbl, "Phase"=w66:dbl)
        n80 = call <vilib>:"Basic Function Generator.vi"("offset"=w79, "sampling info"=w61, "signal type"=w80, "phase"=w76, "amplitude"=w78, "frequency"=w77) -> ("signal out"=w58:waveform(dbl))  [unwired: 3 in, 2 out]
        n81 = call <vilib>:"Basic Function Generator.vi"("offset"=w69, "sampling info"=w60, "signal type"=w70, "phase"=w66, "amplitude"=w68, "frequency"=w67) -> ("signal out"=w54:waveform(dbl))  [unwired: 3 in, 2 out]
        n82 = Build Array(w59, w58) -> (w57:waveform(dbl)[])
        n83 = Build Array(w55, w54) -> (w53:waveform(dbl)[])
        n84 = flat-sequence {
          tunnel: w133 -> [w218]
          tunnel: w132 -> [w219]
          tunnel: w131 -> [w220]
          tunnel: w130 -> [w221]
          tunnel: [w221] -> w191
          tunnel: [w220] -> w190
          tunnel: [w219] -> w189
          tunnel: [w218] -> w188
          tunnel: [w217] -> w187
          tunnel: w129 -> [w217]
          tunnel: [w216] -> w186
          tunnel: w128 -> [w216]
          tunnel: w127 -> [w215]
          tunnel: w126 -> [w214]
          tunnel: [w213] -> w185
          tunnel: [w212] -> w184
          tunnel: w57 -> [w211]
          tunnel: [w211] -> w56
          tunnel: w53 -> [w210]
          tunnel: [w232] -> w183
          tunnel: [w231] -> w182
          tunnel: [w230] -> w181
          tunnel: [w229] -> w180
          tunnel: w191 -> [w232]
          tunnel: w190 -> [w231]
          tunnel: w189 -> [w230]
          tunnel: w188 -> [w229]
          tunnel: w187 -> [w228]
          tunnel: w186 -> [w227]
          tunnel: [w226] -> w179
          tunnel: w185 -> [w226]
          tunnel: [w225] -> w178
          tunnel: w184 -> [w225]
          tunnel: [w224] -> w177
          tunnel: [w223] -> w176
          tunnel: w56 -> [w222]
          tunnel: [w239] -> _
          tunnel: [w240] -> w49
          tunnel: [w241] -> _
          tunnel: [w242] -> w48
          tunnel: [w243] -> _
          tunnel: [w245] -> w51
          tunnel: [w238] -> w160
          tunnel: [w237] -> w159
          tunnel: w183 -> [w246]
          tunnel: w182 -> [w244]
          tunnel: w181 -> [w238]
          tunnel: w180 -> [w237]
          tunnel: w179 -> [w236]
          tunnel: w178 -> [w235]
          tunnel: w177 -> [w234]
          tunnel: w176 -> [w233]
          frame #0 {
            n85 = call-poly <vilib>:"DAQmx Write.vi"("task/channels in"=w214, "data"=w210, "error in"=w215) -> ("task out"=w212:refnum<k21>, "error out"=w213:errorcluster)  [unwired: 10 in, 1 out]
          }
          frame #1 {
            n86 = call-poly <vilib>:"DAQmx Write.vi"("task/channels in"=w227, "data"=w222, "error in"=w228) -> ("task out"=w223:refnum<k21>, "error out"=w224:errorcluster)  [unwired: 10 in, 1 out]
          }
          frame #2 {
            n87 = call <vilib>:"DAQmx Start Task.vi"("task/channels in"=w246, "error in"=w244) -> ("task out"=w245:refnum<k21>, "error out"=w243:errorcluster)  [unwired: 12 in]
            n88 = call <vilib>:"DAQmx Start Task.vi"("task/channels in"=w235, "error in"=w236) -> ("task out"=w242:refnum<k21>, "error out"=w241:errorcluster)  [unwired: 12 in]
            n89 = call <vilib>:"DAQmx Start Task.vi"("task/channels in"=w233, "error in"=w234) -> ("task out"=w240:refnum<k21>, "error out"=w239:errorcluster)  [unwired: 12 in]
          }
        }
        n90 = call <vilib>:"DAQmx Start Task.vi"("task/channels in"=w160, "error in"=w159) -> ("task out"=w52:refnum<k21>)  [unwired: 12 in, 1 out]
        n91 = Build Array(w49, w48) -> (→"AO Task":refnum<k21>[])
        n92 = Build Array(w52, w51) -> (→"AI task":refnum<k21>[])
      }
      frame 2 {
        w312 = 0 ("index")
        n93 = global read "Lock-in Globles.vi" "Multiplication factor"() -> (w316:dbl)
        n94 = case shown="False" "Cancel Button" {
          tunnel: [w346 w362] -> w313
          frame False {
            n95 = Index Array(array="OSC Configuration") -> (element=w349:T7)  [unwired: 1 in]
            n96 = Unbundle By Name(w349) -> ("frequency"=w348:dbl)
            n97 = for {
              tunnel: "OSC Configuration" -> [w352] mode=indexing
              tunnel: w348 -> [w351]
              tunnel: [w350] -> w346 mode=indexing
              i -> [w355]
              n98 = Equal?(x=0, y=w355) -> (x = y?=w353:bool)
              n99 = case shown="False" w353 {
                tunnel: w352 -> [w358 w359]
                tunnel: w351 -> [w357 _]
                tunnel: [w356 w359] -> w350
                frame False {
                  n100 = Bundle By Name(cluster=w358, "frequency"=w357) -> (w356:T7)
                }
                frame True {
                }
              }
            }
            n101 = local write "OSC Configuration"(w346) -> ()
            n102 = global write "Lock-in Globles.vi" "OSC Configuration"(w346) -> ()
          }
          frame True {
            n103 = flat-sequence {
              tunnel: [w365] -> w362
              tunnel: [w364] -> w361
              tunnel: [w363] -> w360
              tunnel: w361 -> [w372]
              tunnel: w360 -> [w371]
              frame #0 {
                n104 = global read "Lock-in Globles.vi" "OSC Configuration"() -> (w364:T4)
                n105 = local read "OSC Configuration"() -> (w365:T4)
                n106 = Subtract(x=w364, y=w365) -> (x-y=w370:T11)
                n107 = Index Array(array=w370, index=0) -> (element=w368:T12)
                n108 = Unbundle(w368) -> ("frequency"=w367:dbl)  [unwired: 4 out]
                n109 = Equal?(x=w367, y=0.0) -> (x = y?=w363:bool)
              }
              frame #1 {
                n110 = case shown="False" w371 {
                  tunnel: w372 -> [w374 w375]
                  frame False {
                    n111 = local write "OSC Configuration"(w374) -> ()
                    n112 = global write "Lock-in Globles.vi" "Reset Lockin"(TRUE ("Reset Lockin")) -> ()
                  }
                  frame True {
                    n113 = local write "OSC Configuration"(w375) -> ()
                  }
                }
              }
            }
          }
        }
        n114 = Index Array(array=w313, index=w312) -> (element=w317:T7)
        n115 = Unbundle By Name(w317) -> ("Amplitude"=w315:dbl)
        n116 = local read "Sampling information"() -> (w251:cluster{"Fs":dbl, "#s":dbl}[])
        n117 = Multiply(x=w315, y=w316) -> (x*y=w314:dbl)
        n118 = Bundle By Name(cluster=w317, "Amplitude"=w314) -> (w311:T7)
        n119 = Replace Array Subset(array=w313, new element=w311, index=w312) -> (w272:T4)
        n120 = Index Array(array=w272, index=1) -> (element=w284:T7)
        n121 = Index Array(array=w272, index=3) -> (element=w268:T7)
        n122 = Index Array(array=w272, index=2) -> (element=w269:T7)
        n123 = Index Array(array=w272) -> (element=w285:T7)  [unwired: 1 in]
        n124 = Unbundle By Name(w269) -> ("Signal Type"=w267:T10, "DC"=w266:dbl, "Amplitude"=w265:dbl, "frequency"=w264:dbl, "Phase"=w263:dbl)
        n125 = Unbundle By Name(w284) -> ("Signal Type"=w278:T10, "DC"=w277:dbl, "Amplitude"=w276:dbl, "frequency"=w275:dbl, "Phase"=w274:dbl)
        n126 = Unbundle By Name(w268) -> ("Signal Type"=w262:T10, "DC"=w261:dbl, "Amplitude"=w260:dbl, "frequency"=w259:dbl, "Phase"=w258:dbl)
        n127 = Unbundle By Name(w285) -> ("Signal Type"=w283:T10, "DC"=w282:dbl, "Amplitude"=w281:dbl, "frequency"=w280:dbl, "Phase"=w279:dbl)
        n128 = Index Array(array=w251, index=1) -> (element=w255:cluster{"Fs":dbl, "#s":dbl})
        n129 = Index Array(array=w251) -> (element=w256:cluster{"Fs":dbl, "#s":dbl})  [unwired: 1 in]
        n130 = call <vilib>:"Basic Function Generator.vi"("offset"=w266, "sampling info"=w255, "signal type"=w267, "phase"=w263, "amplitude"=w265, "frequency"=w264) -> ("signal out"=w254:waveform(dbl))  [unwired: 3 in, 2 out]
        n131 = call <vilib>:"Basic Function Generator.vi"("offset"=w282, "sampling info"=w256, "signal type"=w283, "phase"=w279, "amplitude"=w281, "frequency"=w280) -> ("signal out"=w288:waveform(dbl))  [unwired: 3 in, 2 out]
        n132 = call <vilib>:"Basic Function Generator.vi"("offset"=w261, "sampling info"=w255, "signal type"=w262, "phase"=w258, "amplitude"=w260, "frequency"=w259) -> ("signal out"=w253:waveform(dbl))  [unwired: 3 in, 2 out]
        n133 = call <vilib>:"Basic Function Generator.vi"("offset"=w277, "sampling info"=w256, "signal type"=w278, "phase"=w274, "amplitude"=w276, "frequency"=w275) -> ("signal out"=w287:waveform(dbl))  [unwired: 3 in, 2 out]
        n134 = local read "AI task"() -> (w322:refnum<k21>[])
        n135 = Build Array(w254, w253) -> (w252:waveform(dbl)[])
        n136 = Build Array(w288, w287) -> (w273:waveform(dbl)[])
        n137 = local read "AO Task"() -> (w321:refnum<k21>[])
        n138 = Index Array(array=w322) -> (element=w297:refnum<k21>)  [unwired: 1 in]
        n139 = Index Array(array=w322, index=1) -> (element=w308:refnum<k21>)
        n140 = local read "AI Block Size"() -> (w292:i32)
        n141 = property class="DAQmx Read"(reference=w297) -> (reference out=w296:refnum<k21>, "AvailSampPerChan"=w295:u32)  [unwired: 1 in, 1 out]
        n142 = Index Array(array=w321) -> (element=w307:refnum<k21>)  [unwired: 1 in]
        n143 = Index Array(array=w321, index=1) -> (element=w305:refnum<k21>)
        n144 = Divide(x=w295, y=w292) -> (x/y=w294:dbl)
        n145 = Round Toward +Infinity(x=w294) -> (ceil(x): smallest int >= x=w293:dbl)
        n146 = call-poly <vilib>:"DAQmx Write.vi"("task/channels in"=w307, "data"=w273) -> ()  [unwired: 11 in, 3 out]
        n147 = call-poly <vilib>:"DAQmx Write.vi"("task/channels in"=w305, "data"=w252) -> ()  [unwired: 11 in, 3 out]
        n148 = for {
          N: w293 -> [_]
          tunnel: w308 -> [w332]
          tunnel: w292 -> [w329]
          tunnel: [w328] -> w250
          tunnel: w292 -> [w327]
          tunnel: [w326] -> w304
          tunnel: [w325] -> w302
          tunnel: [w324] -> w249
          tunnel: w296 -> [w323]
          n149 = call-poly <vilib>:"DAQmx Read.vi"("task/channels in"=w323, "number of samples per channel"=w329) -> ("task out"=w330:refnum<k21>, "data"=w324:dbl[][])  [unwired: 11 in, 1 out]
          n150 = call-poly <vilib>:"DAQmx Read.vi"("task/channels in"=w332, "number of samples per channel"=w327) -> ("task out"=w331:refnum<k21>, "data"=w328:dbl[][])  [unwired: 11 in, 1 out]
          n151 = property class="DAQmx Read"(reference=w330) -> ("AvailSampPerChan"=w325:u32)  [unwired: 1 in, 2 out]
          n152 = property class="DAQmx Read"(reference=w331) -> ("AvailSampPerChan"=w326:u32)  [unwired: 1 in, 2 out]
        }
        n153 = local read "AI Buffer Size (s)"() -> (w291:i32)
        n154 = local read "AI Rate"() -> (w290:dbl)
        n155 = Compound Arithmetic op=MULTIPLY(invert w291, invert w290, w302, u32 100 ("value")) -> (w299:dbl)
        n156 = Compound Arithmetic op=MULTIPLY(invert w291, invert w290, w304, u32 100 ("value")) -> (w300:dbl)
        n157 = Max & Min(x=w299, y=w300) -> (max(x,y)=→"Backlog":dbl)  [unwired: 1 out]
        n158 = Build Array (concatenate)(w249, w250) -> (w248:dbl[][])
        "Signal" <- w248
        "Input signal" <- w248
        n159 = case shown="True" "Stream to disk?" {
          tunnel: w248 -> [_ w338]
          frame False {
          }
          frame True {
            w342 = FALSE ("averaging")
            n160 = Index Array(array=w338) -> (element #1=w345:dbl[], element #3=w344:dbl[], element #4=w343:dbl[])  [unwired: 8 in, 1 out]
            n161 = call-poly <vilib>:"Decimate (single shot).vi"("averaging"=w342, "decimating factor"="decimating factor", "X"=w345) -> ("Decimated Array"=w341:dbl[])  [unwired: 7 in, 1 out]
            n162 = call-poly <vilib>:"Decimate (single shot).vi"("averaging"=w342, "decimating factor"="decimating factor", "X"=w344) -> ("Decimated Array"=w340:dbl[])  [unwired: 7 in, 1 out]
            n163 = call-poly <vilib>:"Decimate (single shot).vi"("averaging"=w342, "decimating factor"="decimating factor", "X"=w343) -> ("Decimated Array"=w339:dbl[])  [unwired: 7 in, 1 out]
            n164 = call "Read PPMS T and B.vi"() -> ("Field"=w335:dbl, "Temperature"=w336:dbl, "Time"=w337:dbl)  [unwired: 3 in]
            n165 = Build Array(w341, w340, w339) -> (w334:dbl[][])
            n166 = call "Stream_lock_in_data.vi"("Input signal 2"=w334, "decimating factor"="decimating factor", "Field"=w335, "Temperature"=w336, "Time"=w337) -> ()  [unwired: 4 in]
          }
        }
        n167 = Get Date/Time In Seconds() -> (seconds since 1Jan1904=w309:timestamp)
        n168 = global write "Lock-in Globles.vi" "Input signal"(w248) -> ()
        n169 = global write "Lock-in Globles.vi" "timestamp"(w309) -> ()
      }
      frame 3 {
        w383 = enum32{"Top", "Bottom", "Left", "Right"}."Bottom" ("Tab Location")
        n170 = local read "Cancel Button"() -> (w387:bool)
        n171 = local read "Signal"() -> (w423:dbl[][])
        n172 = case shown="False" w387 {
          tunnel: [w425 w426] -> w388
          frame False {
            n173 = local read "OSC Configuration"() -> (w425:T4)
          }
          frame True {
            n174 = global read "Lock-in Globles.vi" "OSC Configuration"() -> (w426:T4)
          }
        }
        n175 = Array Size(array=w423) -> (size(s)=w422:i32[])
        n176 = local read "AI Block Size"() -> (w377:i32)
        n177 = local read "AI Rate"() -> (w376:dbl)
        n178 = property on="Tab Control 2" class="TabCtl (strict)"("Tab Location"=w383) -> ()  [unwired: 2 in, 2 out]
        n179 = property on="Tab Control" class="TabCtl (strict)"("Tab Location"=w383) -> ()  [unwired: 2 in, 2 out]
        n180 = Index Array(array=w422) -> (element=w421:i32)  [unwired: 1 in]
        n181 = for {
          N: w421 -> [_]
          tunnel: w388 -> [w512] mode=indexing
          tunnel: "Phase&Tc" -> [w505] mode=indexing
          tunnel: [w510] -> w424 mode=indexing
          tunnel: w377 -> [w492]
          tunnel: w376 -> [w491]
          i -> [w495]
          n182 = local read "Results"() -> (w509:dbl[][])
          n183 = Unbundle By Name(w512) -> ("frequency"=w511:dbl)
          n184 = local read "phase log"() -> (w496:dbl[])
          n185 = Unbundle By Name(w505) -> ("Phase"=w507:dbl, "Autophase"=w503:bool)  [unwired: 1 out]
          n186 = Index Array(array=w496, index=w495) -> (element=w497:dbl)
          n187 = call "Reference_new version_1.0.vi"("Phase log in"=w497, "AI Block Size"=w492, "Phase&time"=w505, "Frequency"=w511, "AI Rate"=w491) -> ("Ref out"=w510:T13, "Phase log"=w494:dbl)  [unwired: 3 in]
          n188 = Replace Array Subset(array=w496, new element=w494, index=w495) -> (w493:dbl[])
          n189 = Index Array(array=w509, index (row)=w495, index (col)=3 ("disabled index (col)")) -> (element=w506:dbl)
          n190 = case shown="False" w503 {
            selector: w503 -> [w513 _]
            tunnel: w507 -> [w514 w518]
            tunnel: w506 -> [_ w517]
            tunnel: [w514 w516] -> w504
            tunnel: [w513 FALSE] -> w502
            frame False {
            }
            frame True {
              n191 = Add(x=w518, y=w517) -> (x+y=w516:dbl)
            }
          }
          n192 = local write "phase log"(w493) -> ()
          n193 = Bundle By Name(cluster=w505, "Phase"=w504, "Autophase"=w502, "Set Tc"=FALSE) -> (w500:T14)
          n194 = local read "Phase&Tc"() -> (w501:T5)
          n195 = Replace Array Subset(array=w501, new element=w500, index=w495) -> (w499:T5)
          n196 = local write "Phase&Tc"(w499) -> ()
        }
        n197 = call "Lock-in_dem_mul.vi"("Phase&Tc"="Phase&Tc", "Ref in"=w424, "Signal"=w423) -> ("Demodulation"=w378:dbl[][])  [unwired: 2 in]
        "Results" <- w378
        n198 = for {
          tunnel: w378 -> [w441] mode=indexing
          tunnel: [w440] -> w414 mode=indexing
          shift-right: [w437] -> w391
          shift-left: dbl[] [] -> [w438]
          i -> [w443]
          n199 = Index Array(array="Amplifier Settings", index=w443) -> (element=w442:u16)
          n200 = case shown="1" w442 {
            tunnel: w441 -> [w449 w461 w471 w481]
            tunnel: [w446 w459 w468 w480] -> w440
            tunnel: [w445 w456 w467 w479] -> w439
            frame 0, Default {
              n201 = for {
                N: 3 -> [_]
                tunnel: w449 -> [w455] mode=indexing
                tunnel: [w454] -> w450 mode=indexing
                tunnel: [w452] -> w445
                w453 = u16 0 items=["1 - DDPCA Gain (V/A)", "2 - DDPCA Gain (V/A)", "3 - DLPVA Gain (dB)", "3 - Gain 1", "3 - Gain 2", "3 - AC/DC coupling", "3 - filter", "4 - DLPVA Gain (dB)", "4 - Gain 1", "4 - Gain 2", "4 - AC/DC coupling", "4 - filter"] ("Property")
                n202 = call <userlib>:"PPMS_Femto_TXT_Global_READ.vi"("Property"=w453) -> ("Value"=w452:i32)  [unwired: 1 in, 1 out]
                n203 = Divide(x=w455, y=w452) -> (x/y=w454:dbl)
              }
              n204 = Index Array(array=w449, index=3) -> (element=w447:dbl)
              n205 = Build Array (concatenate)(w450, w447) -> (w446:dbl[])
            }
            frame 1 {
              n206 = for {
                N: 3 -> [_]
                tunnel: w461 -> [w466] mode=indexing
                tunnel: [w465] -> w462 mode=indexing
                tunnel: [w463] -> w456
                w464 = u16 1 items=["1 - DDPCA Gain (V/A)", "2 - DDPCA Gain (V/A)", "3 - DLPVA Gain (dB)", "3 - Gain 1", "3 - Gain 2", "3 - AC/DC coupling", "3 - filter", "4 - DLPVA Gain (dB)", "4 - Gain 1", "4 - Gain 2", "4 - AC/DC coupling", "4 - filter"] ("Property")
                n207 = call <userlib>:"PPMS_Femto_TXT_Global_READ.vi"("Property"=w464) -> ("Value"=w463:i32)  [unwired: 1 in, 1 out]
                n208 = Divide(x=w466, y=w463) -> (x/y=w465:dbl)
              }
              n209 = Index Array(array=w461, index=3) -> (element=w460:dbl)
              n210 = Build Array (concatenate)(w462, w460) -> (w459:dbl[])
            }
            frame 2 {
              n211 = for {
                N: 3 -> [_]
                tunnel: w471 -> [w478] mode=indexing
                tunnel: [w477] -> w472 mode=indexing
                tunnel: [w474] -> w467
                w476 = u16 2 items=["1 - DDPCA Gain (V/A)", "2 - DDPCA Gain (V/A)", "3 - DLPVA Gain (dB)", "3 - Gain 1", "3 - Gain 2", "3 - AC/DC coupling", "3 - filter", "4 - DLPVA Gain (dB)", "4 - Gain 1", "4 - Gain 2", "4 - AC/DC coupling", "4 - filter"] ("Property")
                n212 = call <userlib>:"PPMS_Femto_TXT_Global_READ.vi"("Property"=w476) -> ("Value"=w475:i32)  [unwired: 1 in, 1 out]
                n213 = expression code="10**(x/20)"(w475) -> (w474:i32)
                n214 = Divide(x=w478, y=w474) -> (x/y=w477:dbl)
              }
              n215 = Index Array(array=w471, index=3) -> (element=w470:dbl)
              n216 = Build Array (concatenate)(w472, w470) -> (w468:dbl[])
            }
            frame 3 {
              n217 = for {
                N: 3 -> [_]
                tunnel: w481 -> [w490] mode=indexing
                tunnel: [w489] -> w484 mode=indexing
                tunnel: [w486] -> w479
                w488 = u16 7 items=["1 - DDPCA Gain (V/A)", "2 - DDPCA Gain (V/A)", "3 - DLPVA Gain (dB)", "3 - Gain 1", "3 - Gain 2", "3 - AC/DC coupling", "3 - filter", "4 - DLPVA Gain (dB)", "4 - Gain 1", "4 - Gain 2", "4 - AC/DC coupling", "4 - filter"] ("Property")
                n218 = call <userlib>:"PPMS_Femto_TXT_Global_READ.vi"("Property"=w488) -> ("Value"=w487:i32)  [unwired: 1 in, 1 out]
                n219 = expression code="10**(x/20)"(w487) -> (w486:i32)
                n220 = Divide(x=w490, y=w486) -> (x/y=w489:dbl)
              }
              n221 = Index Array(array=w481, index=3) -> (element=w483:dbl)
              n222 = Build Array (concatenate)(w484, w483) -> (w480:dbl[])
            }
          }
          n223 = Build Array (concatenate)(w438, w439) -> (w437:dbl[])
        }
        "Gains" <- w391
        n224 = local read "Amplifier Settings"() -> (w409:u16[])
        n225 = global write "Lock-in Globles.vi" "Results"(w414) -> ()
        n226 = call "Display.vi"("Results"=w414, "Display"="Display", "Lock-in #"=0 ("index (row)"), "Amplifier Settings"=w409) -> ("Display 1"=w401:string, "Display 2"=w400:string, "Array"=→"Display 1X":dbl[], "Array 2"=→"Display 1Y":dbl[])  [unwired: 3 in]
        n227 = call "Display.vi"("Results"=w414, "Display"="Display", "Lock-in #"=1 ("index (row)"), "Amplifier Settings"=w409) -> ("Display 1"=w399:string, "Display 2"=w398:string, "Array"=→"Display 2X":dbl[], "Array 2"=→"Display 2Y":dbl[])  [unwired: 3 in]
        n228 = call "Display.vi"("Results"=w414, "Display"="Display", "Lock-in #"=2 ("index (row)"), "Amplifier Settings"=w409) -> ("Display 1"=w397:string, "Display 2"=w396:string, "Array"=→"Display 3X":dbl[], "Array 2"=→"Display 3Y":dbl[])  [unwired: 3 in]
        n229 = call "Display.vi"("Results"=w414, "Display"="Display", "Lock-in #"=3 ("index (row)"), "Amplifier Settings"=w409) -> ("Display 1"=w395:string, "Display 2"=w394:string, "Array"=→"Display 4X":dbl[], "Array 2"=→"Display 4Y":dbl[])  [unwired: 3 in]
        n230 = global read "Lock-in Globles.vi" "Stop Lockin"() -> (w386:bool)
        n231 = global read "Lock-in Globles.vi" "Reset Lockin"() -> (w380:bool)
        n232 = case shown="\"Input signals\"" "Tab Control" {
          tunnel: w401 -> [w428 _ _ _ w436]
          tunnel: [w428 w430 w432 w434 w436] -> w390
          tunnel: w400 -> [w427 _ _ _ w435]
          tunnel: [w427 w429 w431 w433 w435] -> w389
          tunnel: w399 -> [_ w430 _ _ _]
          tunnel: w398 -> [_ w429 _ _ _]
          tunnel: w397 -> [_ _ w432 _ _]
          tunnel: w396 -> [_ _ w431 _ _]
          tunnel: w395 -> [_ _ _ w434 _]
          tunnel: w394 -> [_ _ _ w433 _]
          frame "Lock-in #1", Default {
          }
          frame "Lock-in #2" {
          }
          frame "Lock-in #3" {
          }
          frame "Lock-in #4" {
          }
          frame "Input signals" {
          }
        }
        "Display 1" <- w390
        "Display 2" <- w389
        n233 = Or(x=w386, y="stop") -> (x .or. y?=w384:bool)
        n234 = Select(t=4.0 ("f"), s=w384, f=2.0) -> (s? t:f=w382:dbl)
        n235 = Select(t=5.0, s=w380, f=w382) -> (s? t:f=w379:dbl)
      }
      frame 4 {
        n236 = local read "AO Task"() -> (w523:refnum<k21>[])
        n237 = local read "AI task"() -> (w525:refnum<k21>[])
        n238 = flat-sequence {
          tunnel: w525 -> [w537]
          tunnel: [w536] -> w524
          tunnel: w523 -> [w536]
          tunnel: [w535] -> w522
          tunnel: w524 -> [w543]
          tunnel: w522 -> [w542]
          tunnel: [w542] -> w521
          tunnel: [w541] -> w520
          frame #0 {
            n239 = for {
              tunnel: w537 -> [w540] mode=indexing
              tunnel: [w538] -> w535 mode=indexing
              n240 = call <vilib>:"DAQmx Stop Task.vi"("task/channels in"=w540) -> ("task out"=w538:refnum<k21>)  [unwired: 13 in, 1 out]
              n241 = Wait (ms)(milliseconds to wait=u32 50) -> ()  [unwired: 1 out]
            }
          }
          frame #1 {
            n242 = for {
              tunnel: w543 -> [w546] mode=indexing
              tunnel: [w544] -> w541 mode=indexing
              n243 = call <vilib>:"DAQmx Stop Task.vi"("task/channels in"=w546) -> ("task out"=w544:refnum<k21>)  [unwired: 13 in, 1 out]
              n244 = Wait (ms)(milliseconds to wait=u32 50) -> ()  [unwired: 1 out]
            }
          }
        }
        n245 = flat-sequence {
          tunnel: w521 -> [w529]
          tunnel: w520 -> [w528]
          tunnel: [w528] -> w519
          tunnel: w519 -> [w532]
          frame #0 {
            n246 = for {
              tunnel: w529 -> [w531] mode=indexing
              n247 = Wait (ms)(milliseconds to wait=u32 50) -> ()  [unwired: 1 out]
              n248 = call <vilib>:"DAQmx Clear Task.vi"("task in"=w531) -> ()  [unwired: 14 in, 1 out]
            }
          }
          frame #1 {
            n249 = for {
              tunnel: w532 -> [w534] mode=indexing
              n250 = call <vilib>:"DAQmx Clear Task.vi"("task in"=w534) -> ()  [unwired: 14 in, 1 out]
              n251 = Wait (ms)(milliseconds to wait=u32 50) -> ()  [unwired: 1 out]
            }
          }
        }
      }
      frame 5 {
        n252 = local read "AO Task"() -> (w549:refnum<k21>[])
        n253 = local read "AI task"() -> (w550:refnum<k21>[])
        n254 = flat-sequence {
          tunnel: w550 -> [w565]
          tunnel: [w564] -> w553
          tunnel: w549 -> [w564]
          tunnel: [w563] -> w552
          tunnel: w553 -> [w571]
          tunnel: w552 -> [w570]
          tunnel: [w570] -> w548
          tunnel: [w569] -> w547
          frame #0 {
            n255 = for {
              tunnel: w565 -> [w568] mode=indexing
              tunnel: [w566] -> w563 mode=indexing
              n256 = call <vilib>:"DAQmx Stop Task.vi"("task/channels in"=w568) -> ("task out"=w566:refnum<k21>)  [unwired: 13 in, 1 out]
              n257 = Wait (ms)(milliseconds to wait=u32 50) -> ()  [unwired: 1 out]
            }
          }
          frame #1 {
            n258 = for {
              tunnel: w571 -> [w574] mode=indexing
              tunnel: [w572] -> w569 mode=indexing
              n259 = call <vilib>:"DAQmx Stop Task.vi"("task/channels in"=w574) -> ("task out"=w572:refnum<k21>)  [unwired: 13 in, 1 out]
              n260 = Wait (ms)(milliseconds to wait=u32 50) -> ()  [unwired: 1 out]
            }
          }
        }
        n261 = flat-sequence {
          tunnel: w548 -> [w557]
          tunnel: w547 -> [w556]
          tunnel: [w556] -> w551
          tunnel: w551 -> [w560]
          frame #0 {
            n262 = for {
              tunnel: w557 -> [w559] mode=indexing
              n263 = Wait (ms)(milliseconds to wait=u32 50) -> ()  [unwired: 1 out]
              n264 = call <vilib>:"DAQmx Clear Task.vi"("task in"=w559) -> ()  [unwired: 14 in, 1 out]
            }
          }
          frame #1 {
            n265 = for {
              tunnel: w560 -> [w562] mode=indexing
              n266 = call <vilib>:"DAQmx Clear Task.vi"("task in"=w562) -> ()  [unwired: 14 in, 1 out]
              n267 = Wait (ms)(milliseconds to wait=u32 50) -> ()  [unwired: 1 out]
            }
          }
        }
      }
    }
  }
